vi "LuaVIEW Format HTML Function List.vi"(0 "filter":string, 1 "source":string, 5 "names":string[](array[string]), 7 "synopses":string[](array[string]), 9 "docstrings":string[](array[string]), 11 "reentrancy flags":bool[](array[boolean])=[TRUE, FALSE, TRUE, FALSE, TRUE, FALSE, TRUE]) -> (8 "HTML list":string)   [LabVIEW 2012]
doc: "Gernerates a HTML page containing a function index, background information, and a list of function documentations."
uses:
  library/glb_Library Configuration Globals.vi
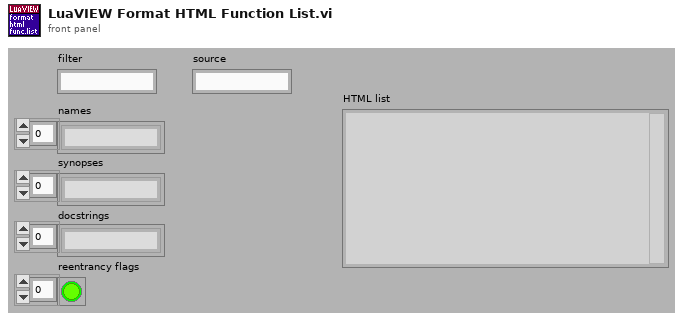
[diagram p1: front panel]
types:
  T1 = enum16{"head", "time/source/filter", "index", "background", "replace < and >", "documentation list", "footer"}
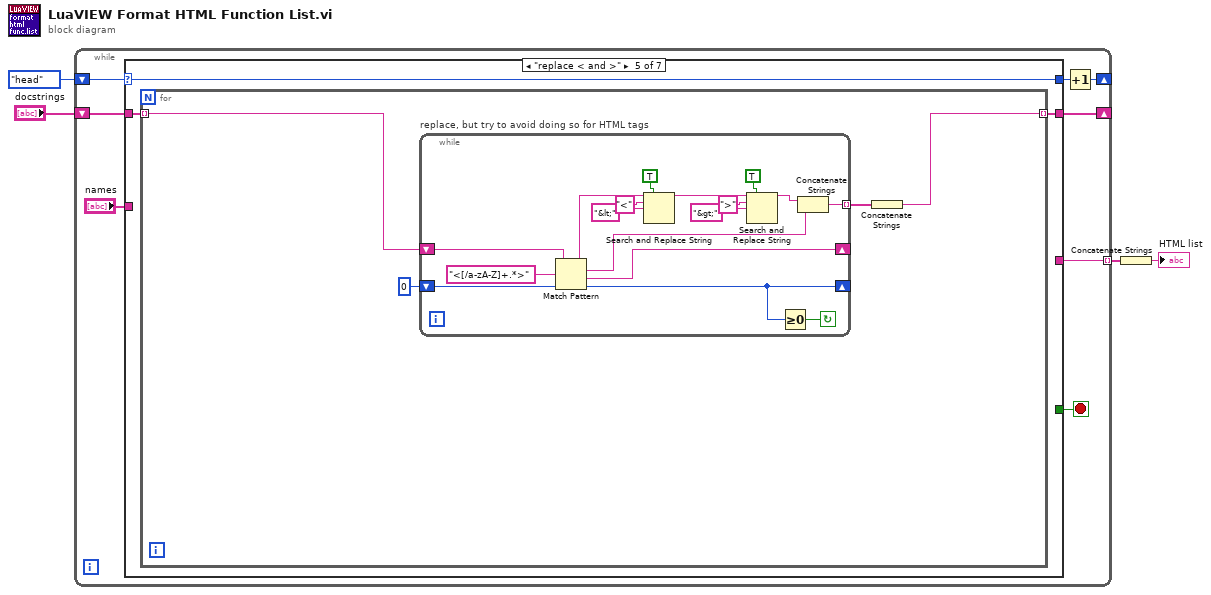
[diagram p0: block diagram]
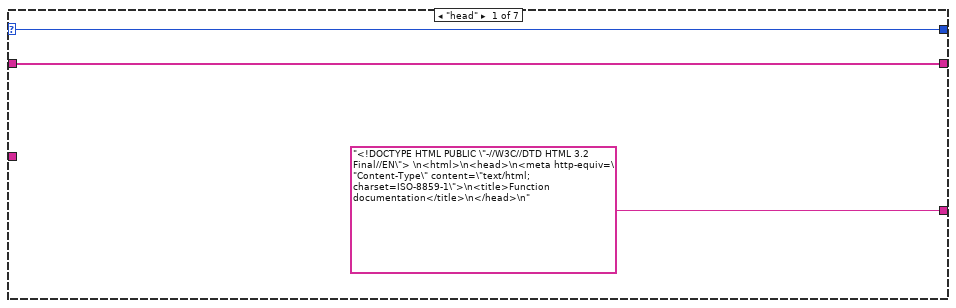
[diagram p2: hidden frame]
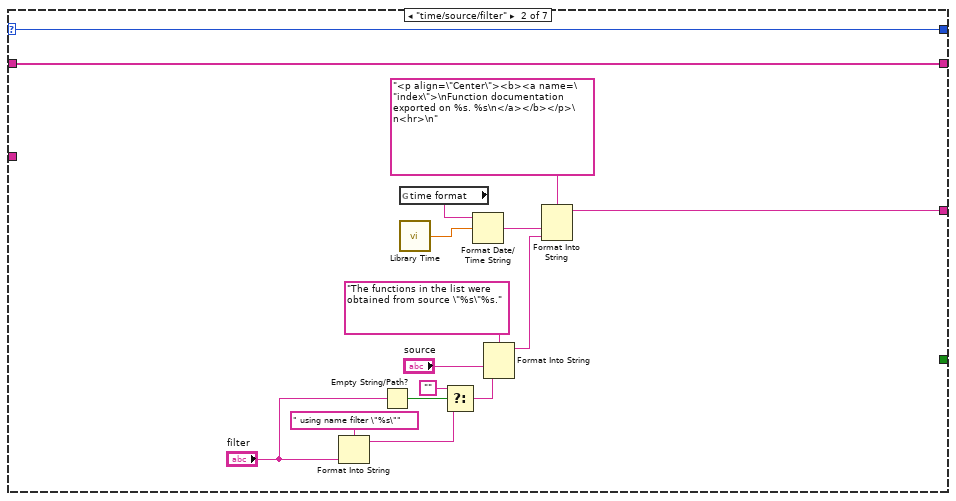
[diagram p3: hidden frame]
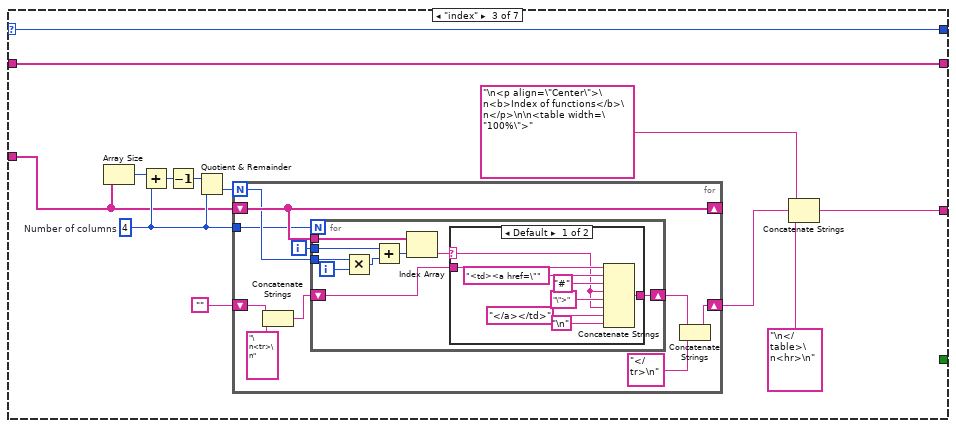
[diagram p4: hidden frame]
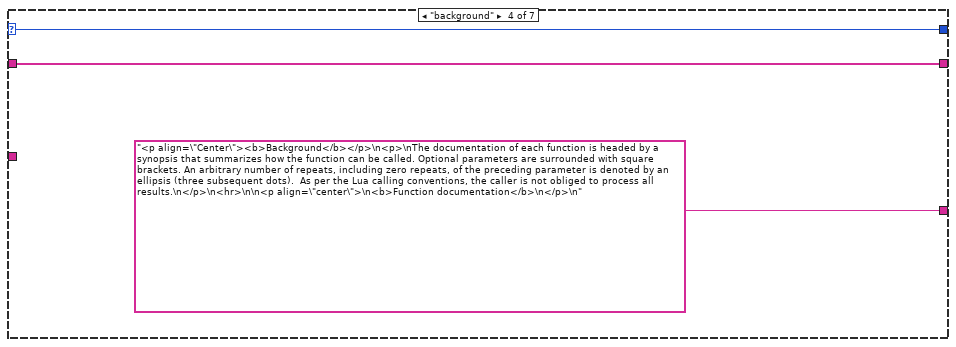
[diagram p6: hidden frame]
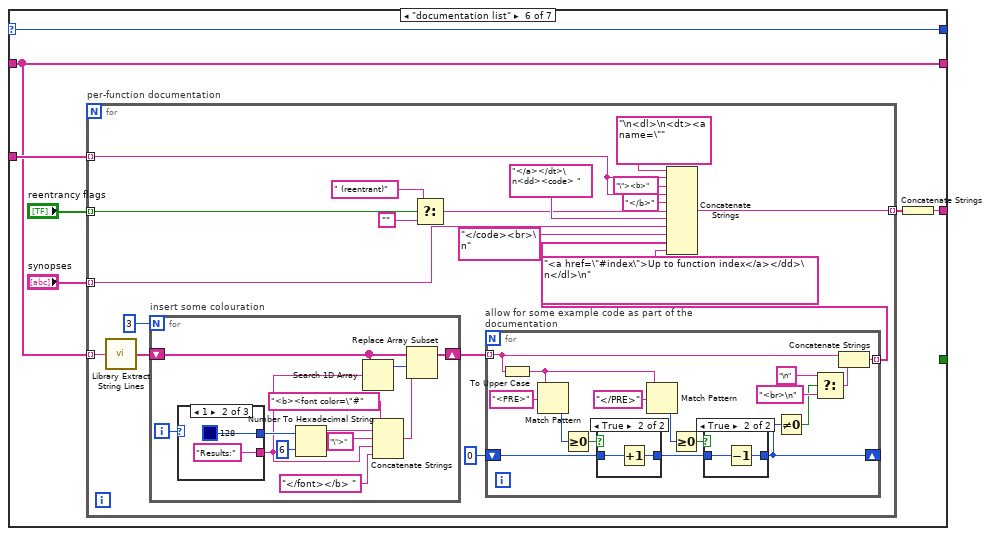
[diagram p7: hidden frame]
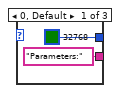
[diagram p10: hidden frame]
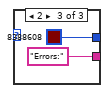
[diagram p11: hidden frame]
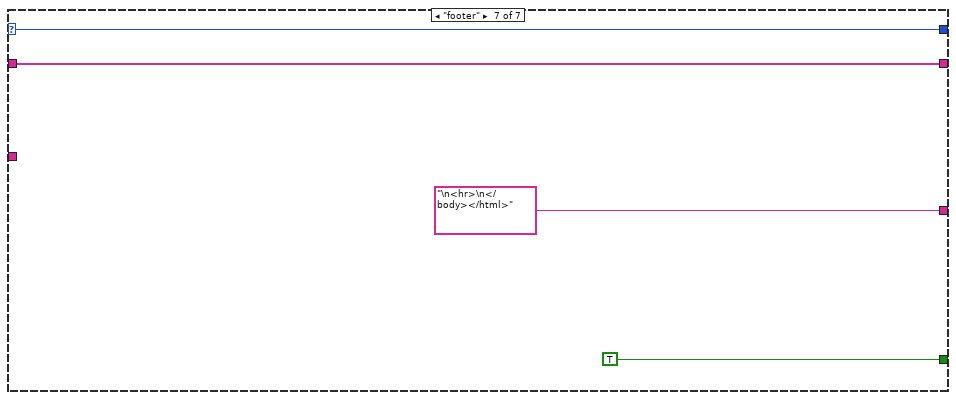
[diagram p12: hidden frame]
diagram:
  n1 = while {
    shift-right: [w8] -> _
    shift-left: T1."head" -> [w10]
    tunnel: [w7] -> w2 mode=indexing
    shift-right: [w5] -> _
    shift-left: "docstrings" -> [w6]
    stop <- w12 stop-if-true
    n2 = case shown="\"replace < and >\"" w10 {
      selector: w10 -> [w15 w24 w44 w75 w78 w106 w168]
      tunnel: [_ _ _ _ _ _ TRUE] -> w12
      tunnel: "names" -> [_ _ w35 _ _ w102 _]
      tunnel: [w15 w24 w44 w75 w78 w106 w168] -> w9
      tunnel: ["<!DOCTYPE HTML PUBLIC \"-//W3C//DTD HTML 3.2 Final//EN\"> \n<html>\n<head>\n<meta http-equiv=\"Content-Type\" content=\"text/html; charset=ISO-8859-1\">\n<title>Function documentation</title>\n</head>\n" w23 w33 "<p align=\"Center\"><b>Background</b></p>\n<p>\nThe documentation of each function is headed by a synopsis that summarizes how the function can be called. Optional parameters are surrounded with square brackets. An arbitrary number of repeats, including zero repeats, of the preceding parameter is denoted by an ellipsis (three subsequent dots).  As per the Lua calling conventions, the caller is not obliged to process all results.\n</p>\n<hr>\n\n<p align=\"center\">\n<b>Function documentation</b>\n</p>\n" ("string") _ w101 "\n<hr>\n</body></html>"] -> w7
      tunnel: w6 -> [w13 w16 w32 w73 w77 w100 w166]
      tunnel: [w13 w16 w32 w73 w76 w100 w166] -> w5
      frame "head" {
      }
      frame "time/source/filter" {
        n3 = Format Into String(format string=" using name filter \"%s\"", "filter") -> (resulting string=w18:string)  [unwired: 2 in, 1 out]
        n4 = Empty String/Path?(string/path="filter") -> (empty?=w21:bool)
        n5 = global read "glb_Library Configuration Globals.vi" "time format"() -> (w26:string)
        n6 = call "Library Time.vi"() -> ("time"=w25:dbl)  [unwired: 1 in]
        n7 = Select(t="", s=w21, f=w18) -> (s? t:f=w20:string)
        n8 = Format Date/Time String(time format string (%c)=w26, seconds (now)=w25) -> (date/time string=w30:string)  [unwired: 1 in]
        n9 = Format Into String(format string="The functions in the list were obtained from source \"%s\"%s." ("time format string (%c)"), "source", w20) -> (resulting string=w28:string)  [unwired: 2 in, 1 out]
        n10 = Format Into String(format string="<p align=\"Center\"><b><a name=\"index\">\nFunction documentation exported on %s. %s\n</a></b></p>\n<hr>\n" ("string"), w30, w28) -> (resulting string=w23:string)  [unwired: 2 in, 1 out]
      }
      frame "index" {
        w38 = 4  # Number of columns
        n11 = Array Size(array=w35) -> (size(s)=w40:i32)
        n12 = Add(x=w40, y=w38) -> (x+y=w39:i32)
        n13 = Decrement(x=w39) -> (x-1=w37:i32)
        n14 = Quotient & Remainder(x=w37, y=w38) -> (floor(x/y)=w36:i32)  [unwired: 1 out]
        n15 = for {
          N: w36 -> [w46]
          shift-right: [w54] -> _
          shift-left: w35 -> [w54]
          shift-right: [w48] -> w41
          shift-left: "" -> [w51]
          tunnel: w38 -> [w45]
          i -> [w53]
          n16 = Concatenate Strings(w51, "\n<tr>\n" ("element")) -> (w52:string)
          n17 = for {
            N: w45 -> [_]
            tunnel: w54 -> [w63]
            tunnel: w46 -> [w61]
            tunnel: w53 -> [w62]
            shift-right: [w56] -> w49
            shift-left: w52 -> [w57]
            i -> [w59]
            n18 = Multiply(x=w61, y=w59) -> (x*y=w60:i32)
            n19 = Add(x=w62, y=w60) -> (x+y=w58:i32)
            n20 = Index Array(array=w63, index=w58) -> (element=w55:string)
            n21 = case shown="Default" w55 {
              selector: w55 -> [w64 _]
              tunnel: w57 -> [w66 w72]
              tunnel: [w65 w72] -> w56
              frame Default {
                n22 = Concatenate Strings(w66, "<td><a href=\"", "#", w64, "\">", w64, "</a></td>", "\n") -> (w65:string)
              }
              frame "" {
              }
            }
          }
          n23 = Concatenate Strings(w49, "</tr>\n" ("string")) -> (w48:string)
        }
        n24 = Concatenate Strings("\n<p align=\"Center\">\n<b>Index of functions</b>\n</p>\n\n<table width=\"100%\">", w41, "\n</table>\n<hr>\n" ("string")) -> (w33:string)
      }
      frame "background" {
      }
      frame "replace < and >" {
        n25 = for {
          tunnel: w77 -> [w81] mode=indexing
          tunnel: [w79] -> w76 mode=indexing
          n26 = while "replace, but try to avoid doing so for HTML tags" {
            shift-right: [w96] -> _
            shift-left: 0 ("offset past match") -> [w98]
            shift-right: [w95] -> _
            shift-left: w81 -> [w94]
            tunnel: [w83] -> w80 mode=indexing
            stop <- w97 continue-if-true
            n27 = Match Pattern(string=w94, regular expression="<[/a-zA-Z]+.*>", offset (0)=w98) -> (before substring=w93:string, match substring=w84:string, after substring=w95:string, offset past match=w96:i32)
            n28 = Search and Replace String(replace all?=TRUE ("replace all? (F)"), input string=w93, search string="<", replace string="&lt;" ("replace string (\"\")")) -> (result string=w87:string)  [unwired: 4 in, 3 out]
            n29 = Search and Replace String(replace all?=TRUE ("replace all? (F)"), input string=w87, search string=">", replace string="&gt;" ("replace string (\"\")")) -> (result string=w85:string)  [unwired: 4 in, 3 out]
            n30 = Greater Or Equal To 0?(x=w96) -> (x >= 0?=w97:bool)
            n31 = Concatenate Strings(w85, w84) -> (w83:string)
          }
          n32 = Concatenate Strings(w80) -> (w79:string)
        }
      }
      frame "documentation list" {
        n33 = for "per-function documentation" {
          tunnel: w100 -> [w111] mode=indexing
          tunnel: "synopses" -> [w110] mode=indexing
          tunnel: "reentrancy flags" -> [w109] mode=indexing
          tunnel: w102 -> [w108] mode=indexing
          tunnel: [w107] -> w105 mode=indexing
          n34 = call "Library Extract String Lines.vi"("multi-line string"=w111) -> ("lines"=w119:string[])  [unwired: 14 in]
          n35 = for "insert some colouration" {
            N: 3 -> [_]
            shift-right: [w156] -> w114
            shift-left: w119 -> [w157]
            i -> [w158]
            n36 = case shown="1" w158 {
              tunnel: ["Parameters:" ("element") "Results:" ("element") "Errors:" ("element")] -> w152
              tunnel: [u32 32768 u32 128 u32 8388608] -> w155
              frame 0, Default {
              }
              frame 1 {
              }
              frame 2 {
              }
            }
            n37 = Number To Hexadecimal String(1:i16 6 ("width (-)"), 2:w155) -> (0:w153:string)
            n38 = Search 1D Array(1D array=w157, element=w152) -> (index of element=w151:i32)  [unwired: 1 in]
            n39 = Concatenate Strings("<b><font color=\"#" ("new element/subarray"), w153, "\">", w152, "</font></b> " ("string")) -> (w159:string)
            n40 = Replace Array Subset(array=w157, new element=w159, index=w151) -> (w156:string[])
          }
          n41 = Select(t=" (reentrant)", s=w109, f="") -> (s? t:f=w118:string)
          n42 = for "allow for some example code as part of the documentation" {
            tunnel: w114 -> [w140] mode=indexing
            tunnel: [w141] -> w112 mode=indexing
            shift-right: [w126] -> _
            shift-left: 0 -> [w132]
            n43 = To Upper Case(1:w140) -> (0:w134:string)
            n44 = Match Pattern(string=w134, regular expression="<PRE>") -> (offset past match=w131:i32)  [unwired: 1 in, 3 out]
            n45 = Greater Or Equal To 0?(x=w131) -> (x >= 0?=w130:bool)
            n46 = case shown="True" w130 {
              tunnel: w132 -> [w145 w147]
              tunnel: [w145 w146] -> w127
              frame False {
              }
              frame True {
                n47 = Increment(x=w147) -> (x+1=w146:i32)
              }
            }
            n48 = Match Pattern(string=w134, regular expression="</PRE>") -> (offset past match=w128:i32)  [unwired: 1 in, 3 out]
            n49 = Greater Or Equal To 0?(x=w128) -> (x >= 0?=w129:bool)
            n50 = case shown="True" w129 {
              tunnel: w127 -> [w142 w144]
              tunnel: [w142 w143] -> w126
              frame False {
              }
              frame True {
                n51 = Decrement(x=w144) -> (x-1=w143:i32)
              }
            }
            n52 = Not Equal To 0?(x=w126) -> (x != 0?=w133:bool)
            n53 = Select(t="\n" ("string"), s=w133, f="<br>\n" ("string")) -> (s? t:f=w135:string)
            n54 = Concatenate Strings(w140, w135) -> (w141:string)
          }
          n55 = Concatenate Strings("\n<dl>\n<dt><a name=\"", w108, "\"><b>", w108, "</b>" ("string"), w118, "</a></dt>\n<dd><code> " ("string"), w110, "</code><br>\n" ("string"), w112, "<a href=\"#index\">Up to function index</a></dd>\n</dl>\n" ("string")) -> (w107:string)
        }
        n56 = Concatenate Strings(w105) -> (w101:string)
      }
      frame "footer" {
      }
    }
    n57 = Increment(x=w9) -> (x+1=w8:T1)
  }
  n58 = Concatenate Strings(w2) -> (→"HTML list":string)
